vi "Link Control References.vi"(8 "error in (no error)":errorcluster, 10 "Control References":T1[](array[typedef]), 11 "Configuration Editor in":refnum<class "Configuration Editor.lvclass">) -> (0 "error out":errorcluster, 3 "Configuration Editor out":refnum<class "Configuration Editor.lvclass">)   [LabVIEW 2023, in "Configuration Editor.lvlib" / "Configuration Editor.lvclass"]
doc: "<b> Link Control References </b>\n<b> Engine Level </b>\nThis is the base abstraction layer. The purpose of this method is to link the control references to the class private data."
uses:
  Library/Configuration Editor.lvclass
  builds/Framework/Engine.lvlibp/Engine/Custom Controls/Control Reference.ctl
  Library/Configuration Editor.lvclass/Configuration Editor.ctl
  builds/Main/Docking.lvlibp/Prime Panel/PrimeDock.lvclass
  builds/Framework/Engine.lvlibp/Engine/Library/Engine.lvclass
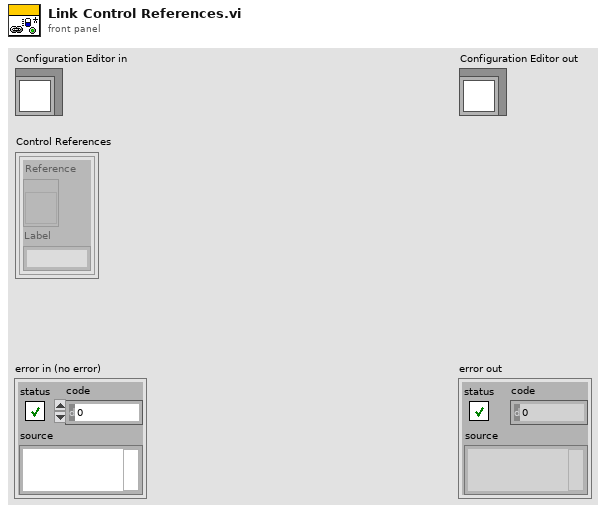
[diagram p1: front panel]
types:
  T1 = typedef "Engine.lvlibp/Engine.lvclass/Control Reference.ctl" = cluster{"Reference":refnum<vi>, "Label":string}
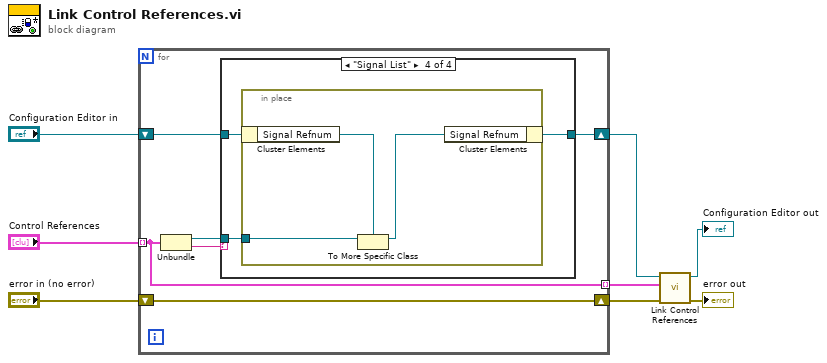
[diagram p0: block diagram]
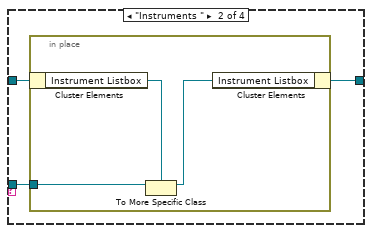
[diagram p3: hidden frame]
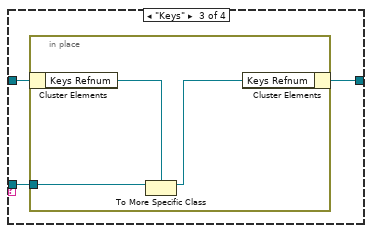
[diagram p4: hidden frame]
diagram:
  n1 = for {
    shift-right: [w9] -> w5
    shift-left: "Configuration Editor in" -> [w10]
    tunnel: "Control References" -> [w13] mode=indexing
    tunnel: [w13] -> w3 mode=indexing
    shift-right: [w14] -> w1
    shift-left: "error in (no error)" -> [w14]
    n2 = Unbundle(w13) -> ("Reference"=w11:refnum<vi>, "Label"=w12:string)
    n3 = case shown="\"Signal List\"" w12 {
      tunnel: w11 -> [_ w16 w22 w28]
      tunnel: w10 -> [w15 w18 w24 w30]
      tunnel: [w15 w17 w23 w29] -> w9
      frame "False", Default {
      }
      frame "Instruments " {
        n4 = in-place {
          in-place-border: w16 -> [w21]
          n5 = in-place-cluster #1(w18) -> ("Instrument Listbox"=w20:refnum<vi>)
          n6 = To More Specific Class(target class=w20, reference=w21) -> (specific class reference=w19:refnum<vi>)  [unwired: 1 in, 1 out]
          n7 = in-place-cluster #1("Instrument Listbox"=w19) -> (w17:refnum<class "Configuration Editor.lvclass">)
        }
      }
      frame "Keys" {
        n8 = in-place {
          in-place-border: w22 -> [w27]
          n9 = in-place-cluster #2(w24) -> ("Keys Refnum"=w26:refnum<vi>)
          n10 = To More Specific Class(target class=w26, reference=w27) -> (specific class reference=w25:refnum<vi>)  [unwired: 1 in, 1 out]
          n11 = in-place-cluster #2("Keys Refnum"=w25) -> (w23:refnum<class "Configuration Editor.lvclass">)
        }
      }
      frame "Signal List" {
        n12 = in-place {
          in-place-border: w28 -> [w33]
          n13 = in-place-cluster #3(w30) -> ("Signal Refnum"=w32:refnum<vi>)
          n14 = To More Specific Class(target class=w32, reference=w33) -> (specific class reference=w31:refnum<vi>)  [unwired: 1 in, 1 out]
          n15 = in-place-cluster #3("Signal Refnum"=w31) -> (w29:refnum<class "Configuration Editor.lvclass">)
        }
      }
    }
  }
  n16 = call-parent "Link Control References.vi"("error in (no error)"=w1, "Control References"=w3, "Engine in"=w5) -> ("error out"=→"error out":errorcluster, "Engine out"=→"Configuration Editor out":refnum<class "Configuration Editor.lvclass">)  [unwired: 7 in]
